vi "Gui_SetupTrapping.vi"(8 "error in (no error)":errorcluster, 10 "Variant for Path":variant, 11 "Variant":variant) -> (0 "error out":errorcluster caption="sortie d'erreur", 3 "Variant Output":variant)   [LabVIEW 2024]
uses:
  controls/SEQUENCE_Inputs.ctl
  controls/EXCIT_Inputs.ctl
  controls/DATA_Inputs.ctl
  controls/TIMING_Inputs.ctl
  controls/PROCESSING_Inputs.ctl
  controls/TRAPPING_Inputs.ctl
  controls/Adiabatic_Waveforms.ctl
  controls/RF_TRAPPING_Inputs.ctl
  controls/EXPERT_Inputs.ctl
  controls/XML_Inputs.ctl
  controls/SOFTWARE_Inputs.ctl
  controls/HSDIO_6541_Inputs.ctl
  <instrlib>/niHSDIO/niHSDIO.llb/niHSDIO_ctl Trigger Source Values (Ring).ctl
  controls/AWG_5421_Inputs.ctl
  <instrlib>/niFgen/niFgen.llb/niFgen_ctl Trigger Source Values (Ring).ctl
  controls/DIGIT_5122_Inputs.ctl
  <instrlib>/niScope/Controls/niScope trigger source.ctl
  controls/AO_6711_Inputs.ctl
  controls/AO_6738_Inputs.ctl
panel:
  in  "CANCEL":bool
  in  "OK":bool
  in  "EXPERT Inputs":T1={"XML Inputs"={"Version Tag Name"="XML_Version", "Version String"="1.0"}, "SOFTWARE Inputs"={"Application Directory"=path "D:/S.O.F.T.S/LABVIEW/PIL", "Software Version"="1.0.0", "Data Path"=path "D:/PIRENEA/DATA", "XML Path"=path "D:/PIRENEA/DATA", "XML File Filter"="*.xml", "XML Saved Path"=path "D:/PIRENEA/DATA/SAVED", "Excit Scripts Path"=path "D:/PIRENEA/EXCIT_SCRIPTS", "Excit Scripts File Filter"="*.txt", "Excit Waveforms Path"=path "D:/PIRENEA/EXCIT_WFMS", "Excit Waveforms File Filter"="*.bin", "Timing Scripts Path"=path "D:/PIRENEA/TIMING_SCRIPTS", "Timing Scripts File Filter"="*.txt", "Timing Waveforms Path"=path "D:/PIRENEA/TIMING_WFMS", "Timing Waveforms File Filter"="*.bin", "Trapping Waveforms Path"=path "D:/PIRENEA/TRAPPING_WFMS", "Trapping Waveforms File Filter"="*.bin"}, "HSDIO 6541 Inputs"={"Resource Name"="HSDIO_6541", "Clock Rate"=1000000.0, "Trigger Source"="PFI0"}, "AWG 5421 Inputs"={"Resource Name"="AWG_5421", "Sample Rate"=10000000.0, "Trigger Type"=2, "Trigger Source"="PFI0", "Waveform Gain"=0.31, "Digital Filter ON"=TRUE}, "DIGIT 5122 Inputs"={"Sample Rate"=10000.0, "Resource Name"="DIGIT_5122", "Channel Name"="0", "Trigger Source"="VAL_EXTERNAL", "Vertical Range"=10.0, "Trigger Level"=3.0}, "AO 6711 Inputs"={"Physical Channels"="AO_6711/ao0:3", "Min Voltage"=-10.0, "Max Voltage"=10.0, "Trigger Source"="/AO_6711/PFI3", "Counter"="AO_6711/ctr0"}, "AO 6738 Inputs"={"Physical Channels"="AO_6738/ao0:3", "Min Voltage"=-10.0, "Max Voltage"=10.0, "Trigger Source"="/AO_6738/PFI2", "Counter"="AO_6738/ctr0"}} {"AO 6738 Inputs"."Max Voltage" min=-10.0 max=10.0; "AO 6738 Inputs"."Min Voltage" min=-10.0 max=10.0; "AWG 5421 Inputs"."Sample Rate" format="%.2p"; "AWG 5421 Inputs"."Trigger Type" items=["None", "Software Edge", "Digital Edge", "Digital Level"]; "AO 6711 Inputs"."Max Voltage" min=-10.0 max=10.0; "AO 6711 Inputs"."Min Voltage" min=-10.0 max=10.0; "HSDIO 6541 Inputs"."Clock Rate" format="%.2p"; "DIGIT 5122 Inputs"."Trigger Level" format="%.2f"; "DIGIT 5122 Inputs"."Vertical Range" format="%.2f"; "DIGIT 5122 Inputs"."Sample Rate" step=65535.0 format="%#_3p"}
  in  "TRAPPING Inputs":T12={"Number of Channels"=4, "Init Values"=[2.0, 9.0, 2.0, 9.0], "Opening Values"=[0.0, 0.0, 0.0, 0.0], "Trapping Values"=[2.0, 9.0, 2.0, 9.0], "Emptying Values"=[-10.0, -10.0, -10.0, -10.0], "Adiabatic ON"=FALSE, "Adiabatic Duration"=100, "Adiabatic Waveforms"=["Adiabatic_None_2_2_2000", "Adiabatic_Ramp_9_0_2000", "Adiabatic_None_2_2_2000", "Adiabatic_RC_9_0_2000"], "Ions Refill ON"=FALSE, "Number of Ions Refills"=1} {"Number of Ions Refills" min=1 max=1000; "Trapping Values" min=-10.0 max=10.0; "Init Values" min=-10.0 max=10.0; "Emptying Values" min=-10.0 max=10.0; "Opening Values" min=-10.0 max=10.0}
  in  "SEQUENCE Inputs":T14={"EXCIT Inputs"={"Number of Excitations"=1, "Script Text"="", "Table of Waveforms"=[]}, "DATA Inputs"={"Record Length"=8192, "Sample Rate"=4.0, "Data Type"=0, "Vertical Range"=0.0, "Acquisition Duration"=100000.0}, "TIMING Inputs"={"Number of Acquisitions "=1, "Number of Accumulations"=1, "Table of Waveforms"=[], "Script Text"=""}, "PROCESSING Inputs"={"Reference Mass"=300.0939, "Cyclotron Freq"=255.727, "Magnetron Freq"=0.001}, "TRAPPING Inputs"={"Number of Channels"=4, "Init Values"=[2.0, 5.0, 5.0, 2.0], "Opening Values"=[0.0, 0.0, 0.0, 0.0], "Trapping Values"=[2.0, 5.0, 5.0, 2.0], "Emptying Values"=[-5.0, -5.0, -5.0, -5.0], "Adiabatic ON"=FALSE, "Adiabatic Duration"=0, "Adiabatic Waveforms"=["Adiabatic_None_2_2_2000.bin", "Adiabatic_Ramp_5_0_2000.bin", "Adiabatic_DoubleRamp_5_0_2000.bin", "Adiabatic_RC_2_0_2000.bin"], "Ions Refill ON"=FALSE, "Number of Ions Refills"=4}, "RF_TRAPPING Inputs"={"Init Values"=[0.0, 1.0, 1.0, 0.0], "Opening Values"=[0.0, -4.0, 1.0, 0.0], "Trapping Values"=[0.0, 1.0, 1.0, 0.0], "Emptying Values"=[0.0, 1.0, -7.0, 0.0], "RF Trap ON"=FALSE, "RF Accums"=1, "Number of Voltages"=4}} {"RF_TRAPPING Inputs"."RF Accums" min=1 max=1000; "RF_TRAPPING Inputs"."Trapping Values" min=-10.0 max=10.0; "RF_TRAPPING Inputs"."Init Values" min=-10.0 max=10.0; "RF_TRAPPING Inputs"."Emptying Values" min=-10.0 max=10.0; "RF_TRAPPING Inputs"."Opening Values" min=-10.0 max=10.0; "TRAPPING Inputs"."Number of Ions Refills" min=1 max=1000; "TRAPPING Inputs"."Trapping Values" min=-10.0 max=10.0; "TRAPPING Inputs"."Init Values" min=-10.0 max=10.0; "TRAPPING Inputs"."Emptying Values" min=-10.0 max=10.0; "TRAPPING Inputs"."Opening Values" min=-10.0 max=10.0; "PROCESSING Inputs"."Magnetron Freq" format="%.5g"; "PROCESSING Inputs"."Cyclotron Freq" format="%.5g"; "PROCESSING Inputs"."Reference Mass" format="%.5g"; "TIMING Inputs"."Number of Accumulations" min=0 max=50 step=1; "TIMING Inputs"."Number of Acquisitions" min=1 max=10 step=1; "DATA Inputs"."Vertical Range" items=["0.2"=0.2, "0.4"=0.4, "1"=1.0, "2"=2.0, "4"=4.0, "10"=10.0]; "DATA Inputs"."Data Type" items=["I16", "DBL"]; "DATA Inputs"."Sample Rate" items=["1 MHz"=1000000.0, "2 MHz"=2000000.0, "5 MHz"=5000000.0, "10 MHz"=10000000.0, "20 MHz"=20000000.0, "25 MHz"=25000000.0, "50 MHz"=50000000.0, "100 MHz"=100000000.0]; "EXCIT Inputs"."Number of Excitations" min=1 max=10}
  # "GO_out (Trap_in_B)"
  # "Gout (Trap_out_B)"
  # "GI_in (Trap_in_A)"
  # "Gin (Trap_out_A)"
  # "RF_V1"
  # "RF_V2"
  # "RF_V3"
  # "RF_V4"
  # "GO_out (Trap_in_B)"
  # "Gout (Trap_out_B)"
  # "GI_in (Trap_in_A)"
  # "Gin (Trap_out_A)"
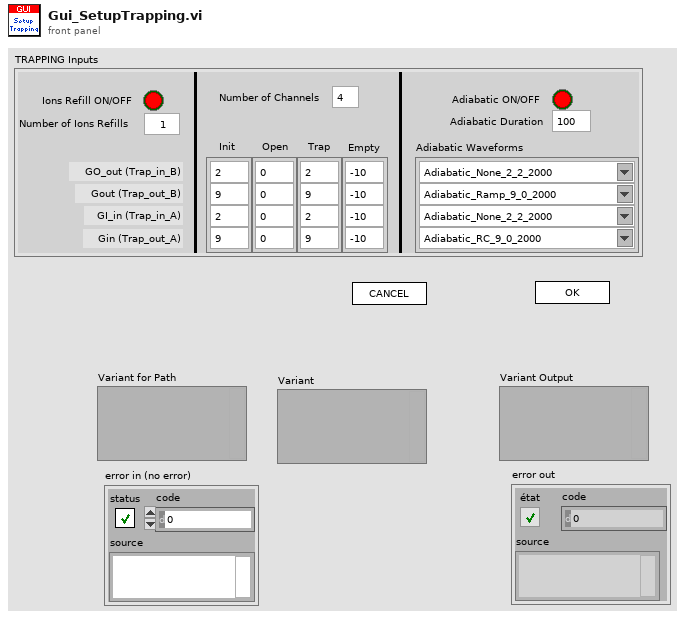
[diagram p1: front panel]
types:
  T1 = typedef "EXPERT_Inputs.ctl" = cluster{"XML Inputs":T2, "SOFTWARE Inputs":T3, "HSDIO 6541 Inputs":T4, "AWG 5421 Inputs":T6, "DIGIT 5122 Inputs":T8, "AO 6711 Inputs":T10, "AO 6738 Inputs":T11}
  T2 = typedef "XML_Inputs.ctl" = cluster{"Version Tag Name":string, "Version String":string}
  T3 = typedef "SOFTWARE_Inputs.ctl" = cluster{"Application Directory":path, "Software Version":string, "Data Path":path, "XML Path":path, "XML File Filter":string, "XML Saved Path":path, "Excit Scripts Path":path, "Excit Scripts File Filter":string, "Excit Waveforms Path":path, "Excit Waveforms File Filter":string, "Timing Scripts Path":path, "Timing Scripts File Filter":string, "Timing Waveforms Path":path, "Timing Waveforms File Filter":string, "Trapping Waveforms Path":path, "Trapping Waveforms File Filter":string}
  T4 = typedef "HSDIO_6541_Inputs.ctl" = cluster{"Resource Name":refnum<k15>, "Clock Rate":dbl, "Trigger Source":T5}
  T5 = typedef "niHSDIO_ctl Trigger Source Values (Ring).ctl" = string
  T6 = typedef "AWG_5421_Inputs.ctl" = cluster{"Resource Name":refnum<k15>, "Sample Rate":dbl, "Trigger Type":u16, "Trigger Source":T7, "Waveform Gain":dbl, "Digital Filter ON":bool}
  T7 = typedef "niFgen_ctl Trigger Source Values (Ring).ctl" = string
  T8 = typedef "DIGIT_5122_Inputs.ctl" = cluster{"Sample Rate":dbl, "Resource Name":refnum<k15>, "Channel Name":string, "Trigger Source":T9, "Vertical Range":dbl, "Trigger Level":dbl}
  T9 = typedef "niScope trigger source.ctl" = string
  T10 = typedef "AO_6711_Inputs.ctl" = cluster{"Physical Channels":tag, "Min Voltage":dbl, "Max Voltage":dbl, "Trigger Source":tag, "Counter":tag}
  T11 = typedef "AO_6738_Inputs.ctl" = cluster{"Physical Channels":tag, "Min Voltage":dbl, "Max Voltage":dbl, "Trigger Source":tag, "Counter":tag}
  T12 = typedef "TRAPPING_Inputs.ctl" = cluster{"Number of Channels":i32, "Init Values":dbl[], "Opening Values":dbl[], "Trapping Values":dbl[], "Emptying Values":dbl[], "Adiabatic ON":bool, "Adiabatic Duration":i32, "Adiabatic Waveforms":T13, "Ions Refill ON":bool, "Number of Ions Refills":i32}
  T13 = typedef "Adiabatic_Waveforms.ctl" = string[]
  T14 = typedef "SEQUENCE_Inputs.ctl" = cluster{"EXCIT Inputs":T15, "DATA Inputs":T16, "TIMING Inputs":T17, "PROCESSING Inputs":T18, "TRAPPING Inputs":T12, "RF_TRAPPING Inputs":T19}
  T15 = typedef "EXCIT_Inputs.ctl" = cluster{"Number of Excitations":i32, "Script Text":string, "Table of Waveforms":string[]}
  T16 = typedef "DATA_Inputs.ctl" = cluster{"Record Length":i32, "Sample Rate":dbl, "Data Type":u8, "Vertical Range":dbl, "Acquisition Duration":dbl}
  T17 = typedef "TIMING_Inputs.ctl" = cluster{"Number of Acquisitions ":i16, "Number of Accumulations":i16, "Table of Waveforms":string[], "Script Text":string}
  T18 = typedef "PROCESSING_Inputs.ctl" = cluster{"Reference Mass":dbl, "Cyclotron Freq":dbl, "Magnetron Freq":dbl}
  T19 = typedef "RF_TRAPPING_Inputs.ctl" = cluster{"Init Values":dbl[], "Opening Values":dbl[], "Trapping Values":dbl[], "Emptying Values":dbl[], "RF Trap ON":bool, "RF Accums":i32, "Number of Voltages":i32}
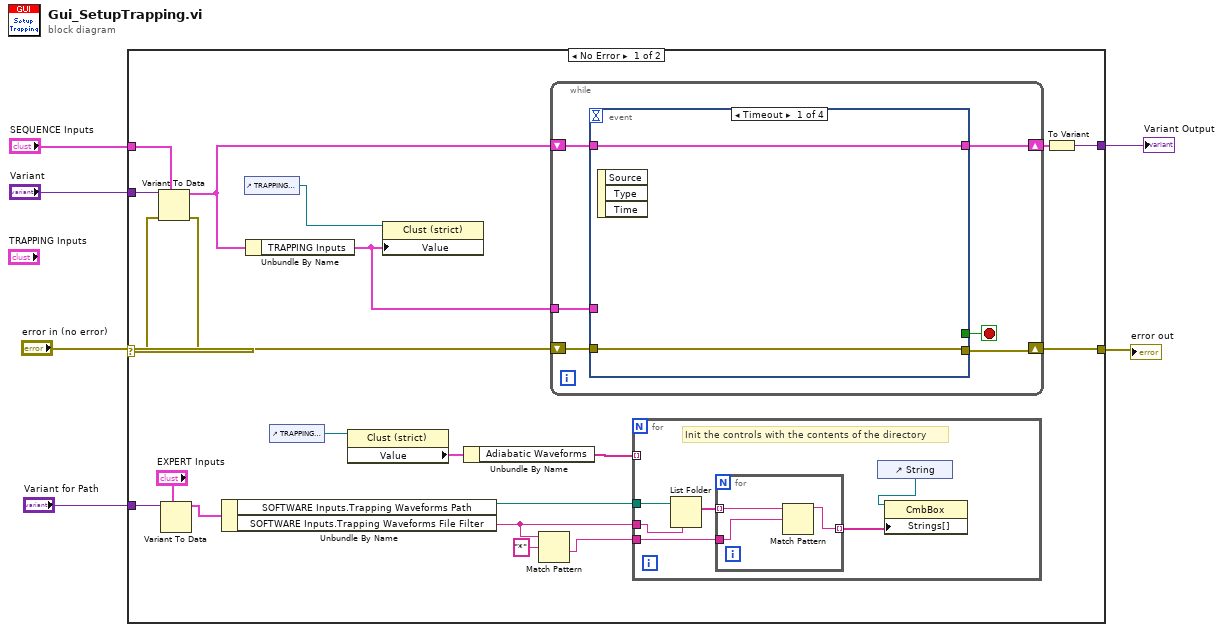
[diagram p0: block diagram]
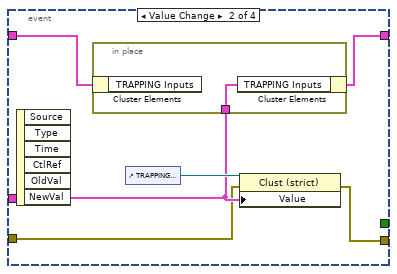
[diagram p2: hidden frame]
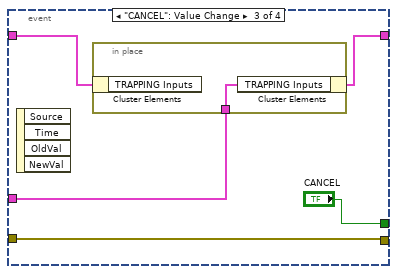
[diagram p3: hidden frame]
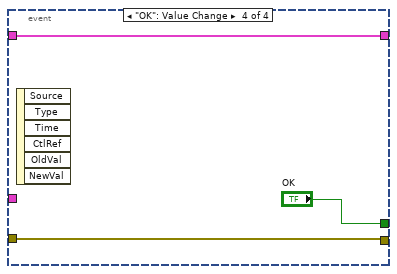
[diagram p4: hidden frame]
diagram:
  n1 = case shown="No Error" "error in (no error)" {
    selector: "error in (no error)" -> [w23 w61]
    tunnel: [w26 w61] -> w5
    tunnel: "Variant" -> [w25 w60]
    tunnel: [w8 w60] -> w3
    tunnel: "Variant for Path" -> [w20 _]
    tunnel: "SEQUENCE Inputs" -> [w11 _]
    frame No Error {
      n2 = Variant To Data(error in=w23, type=w11, Variant=w25) -> (data=w24:T14, error out=w22:errorcluster)
      n3 = Variant To Data(type="EXPERT Inputs", Variant=w20) -> (data=w18:T1)  [unwired: 1 in, 1 out]
      n4 = Unbundle By Name(w18) -> ("SOFTWARE Inputs.Trapping Waveforms Path"=w21:path, "SOFTWARE Inputs.Trapping Waveforms File Filter"=w17:string)
      n5 = control-ref of="TRAPPING Inputs"() -> (w7:refnum<vi>)
      n6 = Unbundle By Name(w24) -> ("TRAPPING Inputs"=w9:T12)
      n7 = control-ref of="TRAPPING Inputs"() -> (w12:refnum<vi>)
      n8 = property class="Clust (strict)"(reference=w12) -> ("Value"=w14:T12)  [unwired: 1 in, 2 out]
      n9 = property class="Clust (strict)"(reference=w7, "Value"=w9) -> ()  [unwired: 1 in, 2 out]
      n10 = Unbundle By Name(w14) -> ("Adiabatic Waveforms"=w13:string[])
      n11 = Match Pattern(string=w17, regular expression="*" ("expression régulière")) -> (after substring=w15:string)  [unwired: 1 in, 3 out]
      n12 = while {
        shift-right: [w29] -> w26
        shift-left: w22 -> [w30]
        shift-right: [w31] -> w10
        shift-left: w24 -> [w32]
        tunnel: w9 -> [w27]
        stop <- w28 stop-if-true
        n13 = event shown="[0] Timeout" {
          selector: _ -> [_ _ _ _]
          dyn-events: _ -> [_ _ _ _]
          timeout: _ -> [_ _ _ _]
          tunnel: w32 -> [w34 w40 w46 w49]
          tunnel: [w34 w39 w45 w49] -> w31
          tunnel: w30 -> [w33 w35 w42 w50]
          tunnel: [w33 w36 w42 w50] -> w29
          tunnel: [_ _ "CANCEL" "OK"] -> w28
          tunnel: w27 -> [_ _ w44 _]
          event Timeout {
            n14 = event-data() -> ()  [unwired: 1 in, 3 out]
          }
          event Value Change {
            n15 = event-data() -> ("NewVal"=w37:T12)  [unwired: 1 in, 5 out]
            n16 = in-place {
              in-place-border: w37 -> [w41]
              n17 = in-place-cluster #1(w40) -> ()  [unwired: 1 out]
              n18 = in-place-cluster #1("TRAPPING Inputs"=w41) -> (w39:T14)
            }
            n19 = control-ref of="TRAPPING Inputs"() -> (w38:refnum<vi>)
            n20 = property class="Clust (strict)"(reference=w38, error in=w35, "Value"=w37) -> (error out=w36:errorcluster)  [unwired: 1 out]
          }
          event "CANCEL": Value Change {
            n21 = event-data() -> ()  [unwired: 1 in, 4 out]
            n22 = in-place {
              in-place-border: w44 -> [w47]
              n23 = in-place-cluster #2(w46) -> ()  [unwired: 1 out]
              n24 = in-place-cluster #2("TRAPPING Inputs"=w47) -> (w45:T14)
            }
          }
          event "OK": Value Change {
            n25 = event-data() -> ()  [unwired: 1 in, 6 out]
          }
        }
      }
      n26 = for {
        tunnel: w21 -> [w54]
        tunnel: w17 -> [w53]
        tunnel: w15 -> [w52]
        tunnel: w13 -> [_] mode=indexing
        # "Init the controls with the contents of the directory"
        n27 = List Folder(path=w54, pattern=w53) -> (filenames=w56:string[])  [unwired: 2 in, 3 out]
        n28 = for {
          tunnel: w56 -> [w59] mode=indexing
          tunnel: [w58] -> w55 mode=indexing
          tunnel: w52 -> [w57]
          n29 = Match Pattern(string=w59, regular expression=w57) -> (before substring=w58:string)  [unwired: 1 in, 3 out]
        }
        n30 = control-ref of="String"() -> (w51:refnum<vi>)
        n31 = property class="CmbBox"(reference=w51, "Strings[]"=w55) -> ()  [unwired: 1 in, 2 out]
      }
      n32 = To Variant(anything=w10) -> (Variant=w8:variant)
    }
    frame Error {
    }
  }
  "error out" <- w5
  "Variant Output" <- w3
